vi "Cheak File.vi"() -> (0 "true":bool)   [LabVIEW 2017]
uses:
  Ctrls/PathChoose.ctl
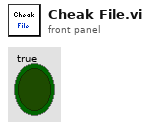
[diagram p1: front panel]
types:
  T1 = typedef "PathChoose.ctl" = enum16{"OperatorLog", "AutoRunLog", "AlmLog", "TestData", "AllTestData", "backup_nvm", "backup_before_flashing"}
  T2 = enum16{"open", "replace", "create", "open or create", "replace or create", "replace or create with confirmation"}
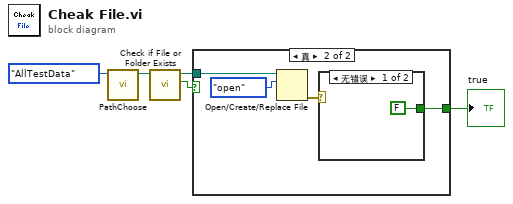
[diagram p0: block diagram]
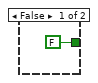
[diagram p2: hidden frame]
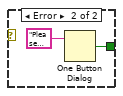
[diagram p3: hidden frame]
diagram:
  n1 = call "PathChoose.vi"(11:PathChoose."AllTestData") -> ("Path_Out"=w1:path)  [unwired: 10 in]
  n2 = call <vilib>:"Check if File or Folder Exists.vi"("path"=w1) -> ("file or folder exists?"=w3:bool, "dup path"=w4:path)  [unwired: 8 in, 1 out]
  n3 = case shown="真" w3 {
    tunnel: w4 -> [_ w9]
    tunnel: [FALSE ("true") w7] -> w2
    frame False {
    }
    frame True {
      n4 = Open/Create/Replace File(file path (use dialog)=w9, operation (0:open)=T2."open") -> (error out=w8:errorcluster)  [unwired: 4 in, 2 out]
      n5 = case shown="无错误" w8 {
        tunnel: [FALSE ("true") w12] -> w7
        frame No Error {
        }
        frame Error {
          n6 = One Button Dialog(message="Please Close The TsetData!") -> (true=w12:bool)  [unwired: 1 in]
        }
      }
    }
  }
  "true" <- w2
